vi "LSCI332 GetAllPar.vi"(6 "error in":errorcluster, 8 "Parameters":T1, 9 "VISA Rsrc":refnum<visa-resource-name>="GPIB0::12::INSTR" caption="Adresse du contrôlleur") -> (0 "error out":errorcluster, 3 "Parameter String":string)   [LabVIEW 2019]
doc: "Ce Vi permet la configuration des limites de contrôles ainsi que la gestion des paramètres de stabilisation. À l'ouverture, le VI lit et retourne les paramètres actuels."
uses:
  <userlib>/LSCI 332 V2/GetAllPAr States.ctl
panel:
  out "Window %":u16
  out "Curve Number":u32
  out "Filter Points":u16
  out "Filtering":bool
  out "Compensation":bool
  out "Sensor Type":T2(ring)
  out "Résistance":u16=50 caption="Résistance Chauffage"
  out "HeatUnits":u32(ring)=1 caption="Heater Units" items=["Current"=1, "Power"=2]
  out "ManOutput":dbl caption="Manual Output %" format="%#.2g"
  out "HtrRange":u16(ring) caption="Échelle de chauffage" items=["Off", "Low (.5W)", "Med (5W)", "High (50W)"]
  out "RampPar":cluster{"Rampe Activée":bool, "RateVal":dbl} caption="Paramètres de Rampe" {"RateVal" step=0.1}
  out "PID":cluster{"P":dbl, "I":dbl, "D":u32}={"P"=1000.0, "I"=0.0, "D"=0} caption="Paramètres PID" {"D" max=1000 step=1; "I" min=0.0 max=1000.0 step=0.1 format="%#.1f"; "P" min=0.0 max=1000.0 step=0.1 format="%#.1f"}
  out "SetPoint":dbl caption="Consigne"
  out "Mode":u32(ring)=1 caption="Mode de Contrôle" items=["Manual PID"=1, "Zone"=2, "Open Loop"=3, "AutoTune PID"=4, "AutoTune PI"=5, "AutoTune P"=6]
  out "PowerUp":bool caption="Contrôle actif \nau démarrage"
  out "Units":u32(ring)=1 caption="Setpoint Units" items=["Kelvin"=1, "Celsius"=2, "Sensor Units"=3]
  out "Input":u32(ring) caption="Entrée de\nTempérature" items=["A", "B"]
  # "Paramètres de la boucle de contrôle"
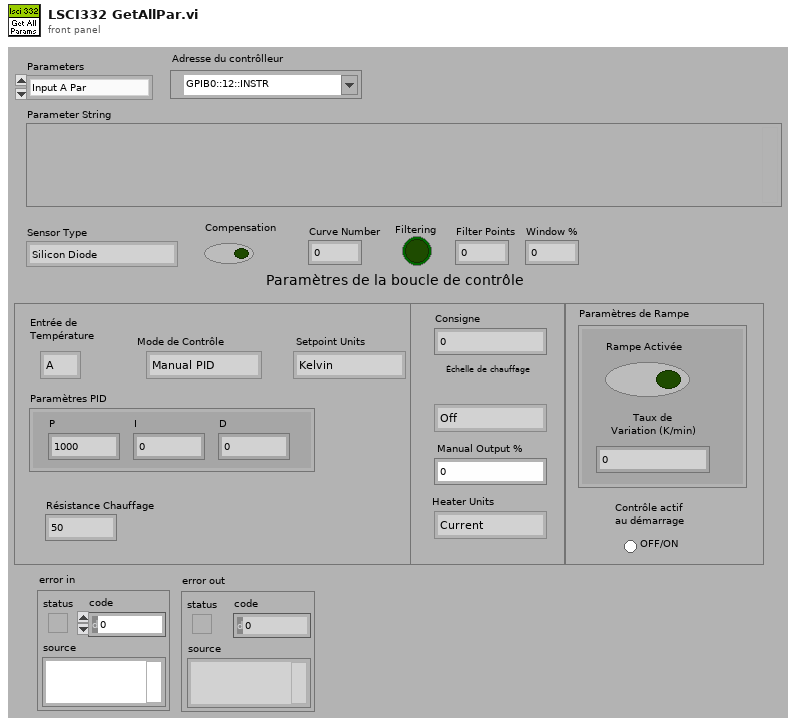
[diagram p1: front panel]
types:
  T1 = typedef "GetAllPAr States.ctl" = enum16{"Input A Par", "Input B Par", "Heater Params", "Loop 1 Par", "Loop 2 Par", "All"}
  T2 = enum16{"Silicon Diode", "GaAlAs", "100 Ohms Platinum/250", "100 Ohms Platinum/500", "1000 Ohms Platinum", "NTC RTD", "Thermocouple 25mv", "Thermocouple 50mv", "2.5V 1mA", "7.5V 1mA"}
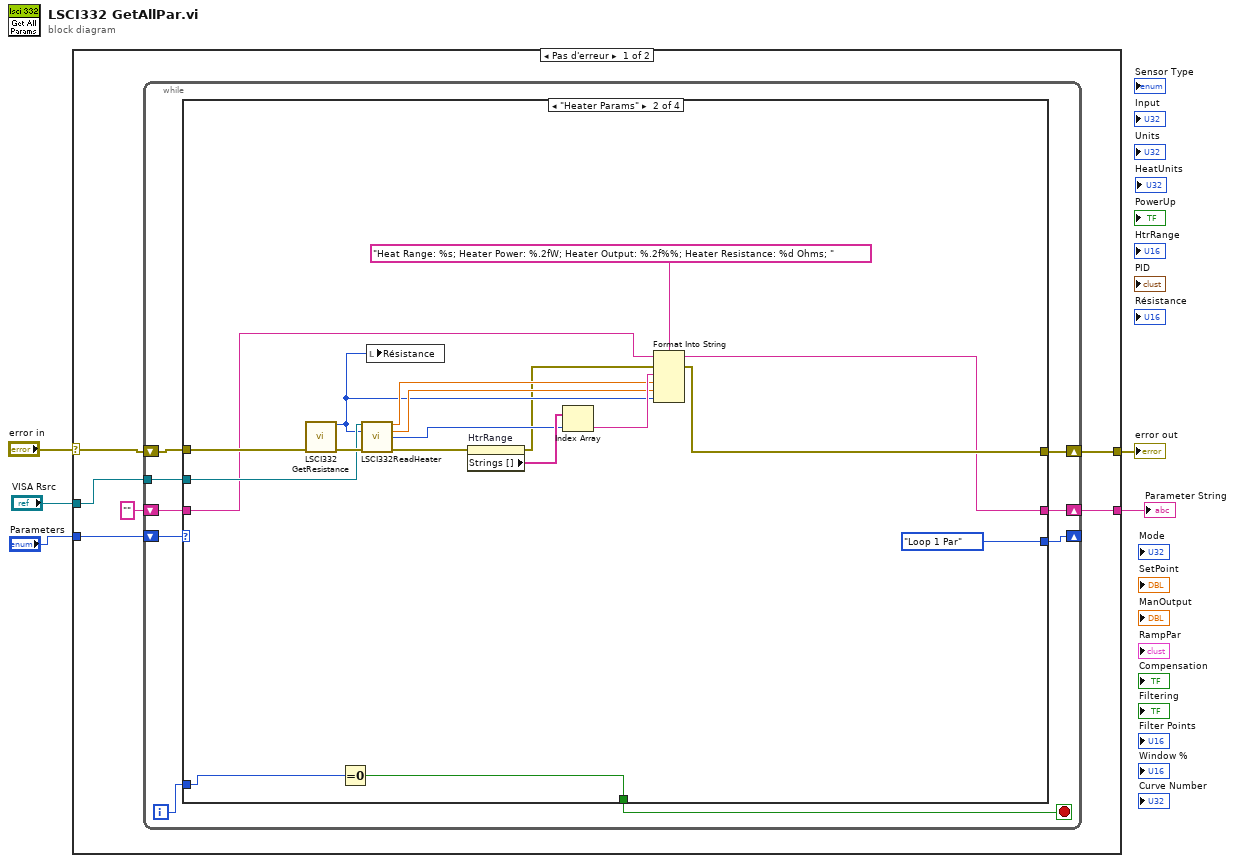
[diagram p0: block diagram]
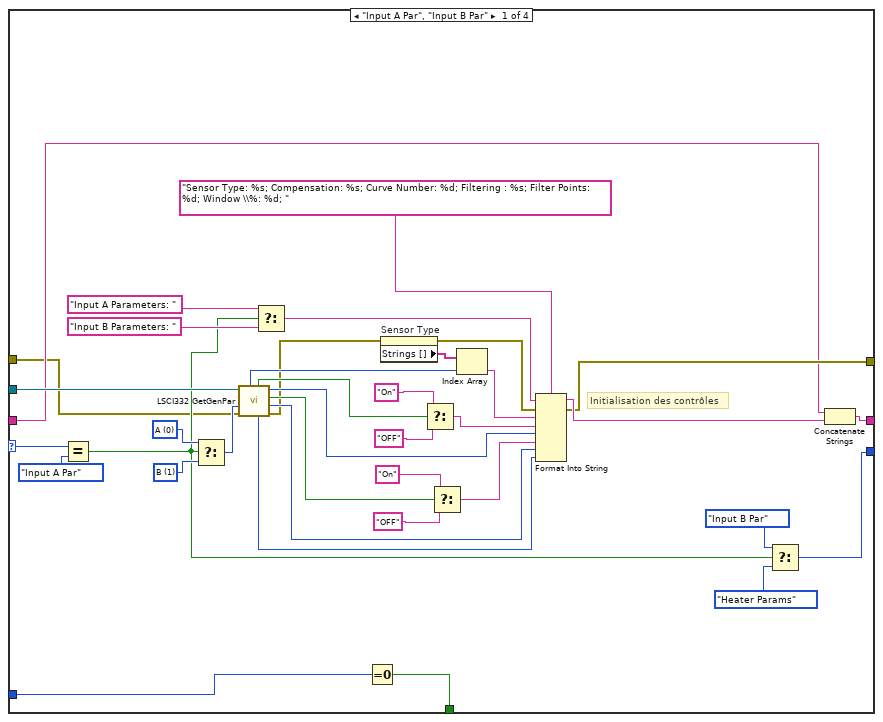
[diagram p2: hidden frame]
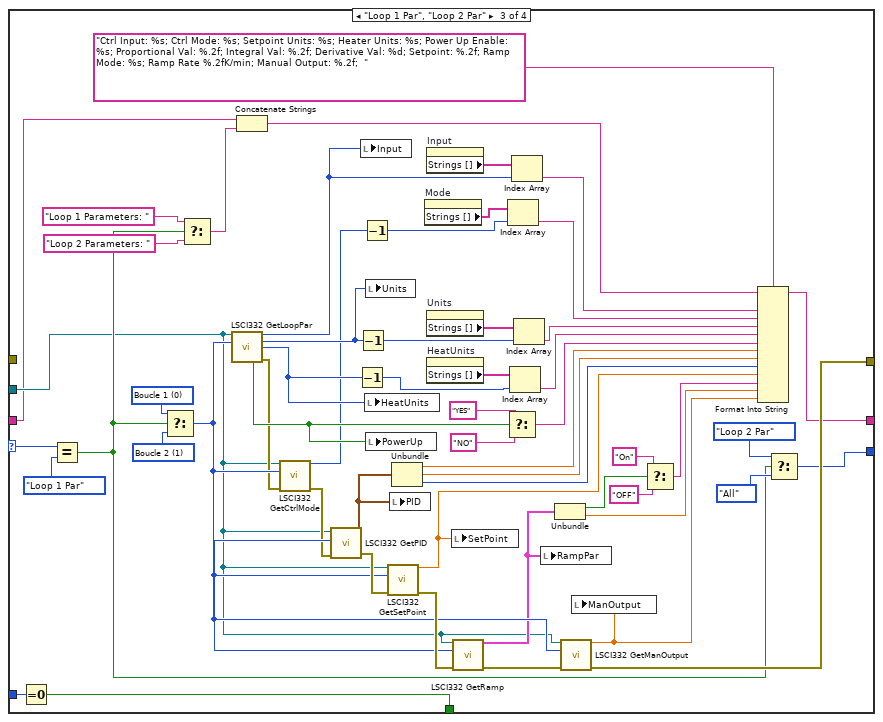
[diagram p3: hidden frame]
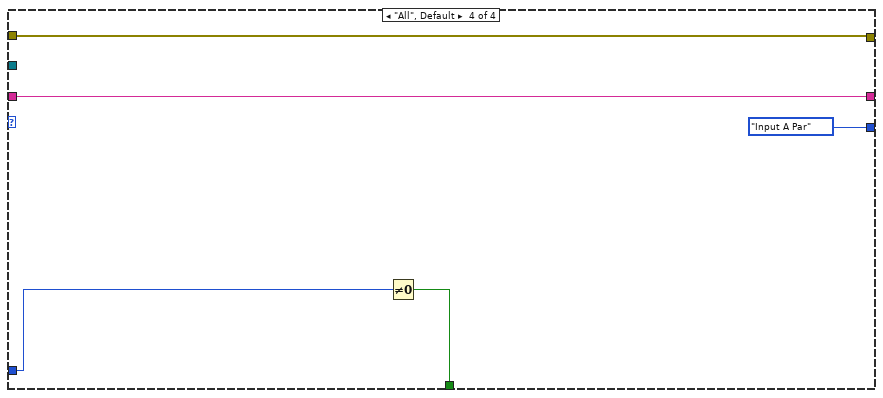
[diagram p4: hidden frame]
diagram:
  n1 = case shown="Pas d'erreur" "error in" {
    selector: "error in" -> [w8 w137]
    tunnel: [w7 w137] -> w4
    tunnel: "VISA Rsrc" -> [w11 _]
    tunnel: "Parameters" -> [w10 _]
    tunnel: [w6 _] -> w1
    frame No Error {
      n2 = while {
        tunnel: w11 -> [w20]
        shift-right: [w18] -> _
        shift-left: w10 -> [w19]
        shift-right: [w17] -> w6
        shift-left: "" -> [w14]
        shift-right: [w13] -> w7
        shift-left: w8 -> [w12]
        i -> [w16]
        stop <- w15 stop-if-true
        n3 = case shown="\"Heater Params\"" w19 {
          selector: w19 -> [w41 _ w126 _]
          tunnel: w20 -> [w57 w72 w82 _]
          tunnel: [w31 GetAllPAr_States."Loop 1 Par" w119 GetAllPAr_States."Input A Par"] -> w18
          tunnel: [w23 w58 w79 w134] -> w17
          tunnel: w16 -> [w35 w74 w129 w136]
          tunnel: [w34 w73 w128 w135] -> w15
          tunnel: w14 -> [w22 w59 w81 w134]
          tunnel: [w24 w60 w122 w132] -> w13
          tunnel: w12 -> [w21 w67 _ w132]
          frame "Input A Par", "Input B Par" {
            w38 = u32 1 items=["A", "B"] ("Input")
            w40 = u32 0 items=["A", "B"] ("Input")
            # "Initialisation des contrôles"
            n4 = Equal?(x=w41, y=GetAllPAr_States."Input A Par") -> (x = y?=w28:bool)
            n5 = Select(t=w40, s=w28, f=w38) -> (s? t:f=w37:u32)
            n6 = call <userlib>:"LSCI332 GetGenPar.vi"("error in (no error)"=w21, "Input"=w37, "VISA Rsrc"=w57) -> ("error out"=w26:errorcluster, "Filter Points"=w43:u16, "Filtering"=w45:bool, "Curve Number"=w48:u32, "Window %"=w42:u16, "Compensation"=w52:bool, "Sensor Type"=w55:T2)  [unwired: 2 in]
            n7 = Select(t="Input A Parameters: ", s=w28, f="Input B Parameters: ") -> (s? t:f=w27:string)
            n8 = Equal To 0?(x=w35) -> (x = 0?=w34:bool)
            n9 = property on="Sensor Type" class="Énum (strict)"(error in=w26) -> (error out=w25:errorcluster, "Strings []"=w56:string[])  [unwired: 1 in, 1 out]
            n10 = Select(t="On", s=w52, f="OFF") -> (s? t:f=w49:string)
            n11 = Select(t="On", s=w45, f="OFF") -> (s? t:f=w44:string)
            n12 = Index Array(array=w56, index=w55) -> (element=w53:string)
            n13 = Format Into String(format string="Sensor Type: %s; Compensation: %s; Curve Number: %d; Filtering : %s; Filter Points: %d; Window \\%: %d; " ("chaîne de format"), initial string=w27, error in=w25, w53, w49, w48, w44, w43, w42) -> (resulting string=w36:string, error out=w24:errorcluster)
            n14 = Select(t=GetAllPAr_States."Input B Par", s=w28, f=GetAllPAr_States."Heater Params") -> (s? t:f=w31:T1)
            n15 = Concatenate Strings(w22, w36) -> (w23:string)
          }
          frame "Heater Params" {
            n16 = call <userlib>:"LSCI332 GetResistance.vi"("error in"=w67) -> ("Résistance"=w62:u16, "error out"=w75:errorcluster)  [unwired: 13 in]
            n17 = Equal To 0?(x=w74) -> (x = 0?=w73:bool)
            n18 = call <userlib>:"LSCI332ReadHeater.vi"("VISA Rsrc"=w72, "Résistance"=w62, "error in"=w75) -> ("Puissance(W)"=w64:dbl, "Puissance(%)"=w63:dbl, "Échelle"=w68:u16, "error out"=w70:errorcluster)  [unwired: 9 in]
            n19 = local write "Résistance"(w62) -> ()
            n20 = property on="HtrRange" class="MDér (strict)"(error in=w70) -> (error out=w61:errorcluster, "Strings []"=w69:string[])  [unwired: 1 in, 1 out]
            n21 = Index Array(array=w69, index=w68) -> (element=w66:string)
            n22 = Format Into String(format string="Heat Range: %s; Heater Power: %.2fW; Heater Output: %.2f%%; Heater Resistance: %d Ohms; " ("chaîne de format"), initial string=w59, error in=w61, w66, w64, w63, w62) -> (resulting string=w58:string, error out=w60:errorcluster)
          }
          frame "Loop 1 Par", "Loop 2 Par" {
            w123 = u32 1 items=["Boucle 1", "Boucle 2"] ("Boucle(1)")
            w124 = u32 0 items=["Boucle 1", "Boucle 2"] ("Boucle(1)")
            n23 = Equal To 0?(x=w129) -> (x = 0?=w128:bool)
            n24 = Equal?(x=w126, y=GetAllPAr_States."Loop 1 Par") -> (x = y?=w112:bool)
            n25 = Select(t=w124, s=w112, f=w123) -> (s? t:f=w96:u32)
            n26 = Select(t="Loop 1 Parameters: ", s=w112, f="Loop 2 Parameters: ") -> (s? t:f=w80:string)
            n27 = call <userlib>:"LSCI332 GetLoopPar.vi"("VISA Rsrc"=w82, "Boucle(1)"=w96) -> ("Input"=w116:u32, "Units"=w115:u32, "HeatUnits"=w113:u32, "PowerUp"=w107:bool, "error out"=w95:errorcluster)  [unwired: 9 in]
            n28 = Concatenate Strings(w81, w80) -> (w78:string)
            n29 = call <userlib>:"LSCI332 GetCtrlMode.vi"("VISA Rsrc"=w82, "Boucle(1)"=w96, "error in (no error)"=w95) -> ("Mode"=w92:u32, "error out"=w94:errorcluster)  [unwired: 11 in]
            n30 = call <userlib>:"LSCI332 GetPID.vi"("error in (no error)"=w94, "Boucle(1)"=w96, "VISA Rsrc"=w82) -> ("error out"=w130:errorcluster, "Paramètres PID"=w101:cluster{"P":dbl, "I":dbl, "D":i32})  [unwired: 6 in]
            n31 = Decrement(x=w113) -> (x-1=w110:u32)
            n32 = Decrement(x=w115) -> (x-1=w111:u32)
            n33 = local write "Input"(w116) -> ()
            n34 = Decrement(x=w92) -> (x-1=w89:u32)
            n35 = local write "HeatUnits"(w113) -> ()
            n36 = local write "Units"(w115) -> ()
            n37 = local write "PowerUp"(w107) -> ()
            n38 = call <userlib>:"LSCI332 GetSetPoint.vi"("VISA Rsrc"=w82, "Boucle(1)"=w96, "error in (no error)"=w130) -> ("SetPoint"=w97:dbl, "error out"=w131:errorcluster)  [unwired: 11 in]
            n39 = local write "PID"(w101) -> ()
            n40 = Unbundle(w101) -> ("P"=w100:dbl, "I"=w99:dbl, "D"=w98:i32)
            n41 = property on="Mode" class="MDér (strict)"() -> ("Strings []"=w91:string[])  [unwired: 2 in, 2 out]
            n42 = property on="Input" class="MDér (strict)"() -> ("Strings []"=w118:string[])  [unwired: 2 in, 2 out]
            n43 = property on="Units" class="MDér (strict)"() -> ("Strings []"=w117:string[])  [unwired: 2 in, 2 out]
            n44 = property on="HeatUnits" class="MDér (strict)"() -> ("Strings []"=w114:string[])  [unwired: 2 in, 2 out]
            n45 = local write "SetPoint"(w97) -> ()
            n46 = call <userlib>:"LSCI332 GetRamp.vi"("VISA Rsrc"=w82, "Boucle(1)"=w96, "error in (no error)"=w131) -> ("Paramètres de Rampe"=w88:cluster{"Rampe activée":bool, "RateVal":dbl}, "error out"=w77:errorcluster)  [unwired: 11 in]
            n47 = Select(t="YES", s=w107, f="NO") -> (s? t:f=w102:string)
            n48 = Index Array(array=w91, index=w89) -> (element=w90:string)
            n49 = Index Array(array=w114, index=w110) -> (element=w103:string)
            n50 = Index Array(array=w118, index=w116) -> (element=w104:string)
            n51 = Index Array(array=w117, index=w111) -> (element=w93:string)
            n52 = local write "RampPar"(w88) -> ()
            n53 = Unbundle(w88) -> ("Rampe activée"=w85:bool, "RateVal"=w83:dbl)
            n54 = call <userlib>:"LSCI332 GetManOutput.vi"("VISA Rsrc"=w82, "Boucle(1)"=w96, "error in"=w77) -> ("ManOutput"=w76:dbl, "error out"=w122:errorcluster)  [unwired: 11 in]
            n55 = local write "ManOutput"(w76) -> ()
            n56 = Select(t="On", s=w85, f="OFF") -> (s? t:f=w84:string)
            n57 = Format Into String(format string="Ctrl Input: %s; Ctrl Mode: %s; Setpoint Units: %s; Heater Units: %s; Power Up Enable: %s; Proportional Val: %.2f; Integral Val: %.2f; Derivative Val: %d; Setpoint: %.2f; Ramp Mode: %s; Ramp Rate %.2fK/min; Manual Output: %.2f;  " ("chaîne de format"), initial string=w78, w104, w90, w93, w103, w102, w100, w99, w98, w97, w84, w83, w76) -> (resulting string=w79:string)  [unwired: 1 in, 1 out]
            n58 = Select(t=GetAllPAr_States."Loop 2 Par", s=w112, f=GetAllPAr_States."All") -> (s? t:f=w119:T1)
          }
          frame "All", Default {
            n59 = Not Equal To 0?(x=w136) -> (x != 0?=w135:bool)
          }
        }
      }
    }
    frame Error {
    }
  }
  "error out" <- w4
  "Parameter String" <- w1
